vi "SetByteOrder.vi"(8 "error in (no error)":errorcluster, 10 "byte order (0:big-endian, network order)":T1(ring), 11 "Gaze in":refnum<class "Gaze.lvclass">) -> (0 "error out":errorcluster, 3 "Gaze out":refnum<class "Gaze.lvclass">)   [LabVIEW 2020, in "Gaze.lvclass"]
uses:
  Gaze.lvclass
  Gaze.lvclass/Gaze.ctl
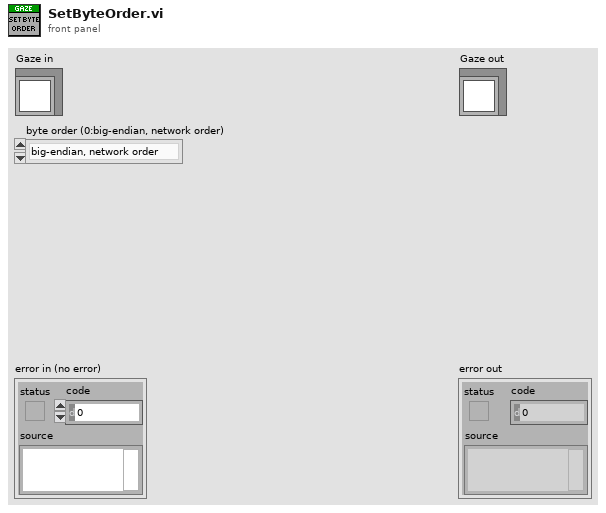
[diagram p1: front panel]
types:
  T1 = enum16{"big-endian, network order", "native, host order", "little-endian"}
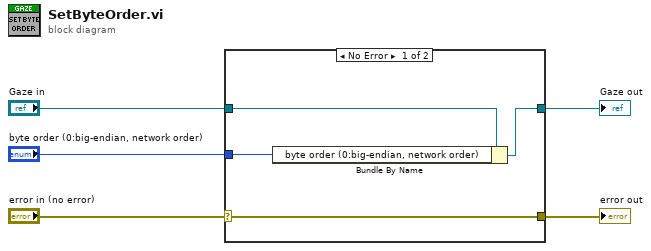
[diagram p0: block diagram]
diagram:
  n1 = case shown="No Error" "error in (no error)" {
    selector: "error in (no error)" -> [w9 w11]
    tunnel: [w9 w11] -> w4
    tunnel: [w7 w10] -> w2
    tunnel: "Gaze in" -> [w8 w10]
    tunnel: "byte order (0:big-endian, network order)" -> [w6 _]
    frame No Error {
      n2 = Bundle By Name(cluster=w8, "byte order (0:big-endian, network order)"=w6) -> (w7:refnum<class "Gaze.lvclass">)
    }
    frame Error {
    }
  }
  "error out" <- w4
  "Gaze out" <- w2
